vi "Handshake.vi"(8 "error in (no error)":errorcluster, 11 "dotNET SSL Socket in":refnum<class "dotNET SSL Server.lvclass">) -> (0 "error out":errorcluster, 3 "dotNET SSL Socket out":refnum<class "dotNET SSL Server.lvclass">)   [LabVIEW 2013, in "dotNET SSL Socket.lvlib" / "dotNET SSL Server.lvclass"]
uses:
  dotNET SSL Server/dotNET SSL Server.lvclass
  dotNET SSL Socket.lvclass/dotNET SSL Socket.ctl
  dotNET SSL Server/dotNET SSL Server.lvclass/dotNET SSL Server.ctl
  Read SSLStream.vi
  Read PFX Certificate.vi
  Read PFX Password.vi
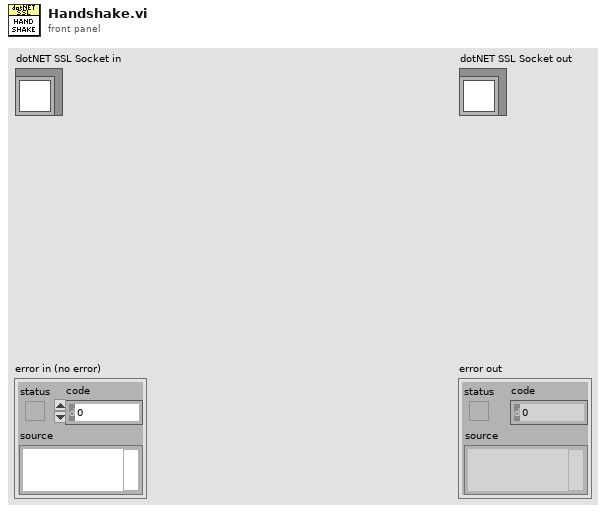
[diagram p1: front panel]
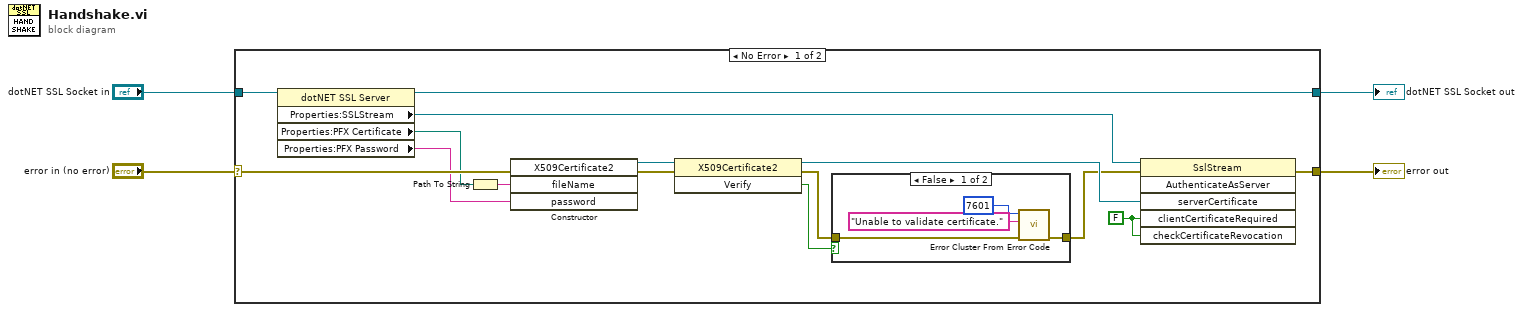
[diagram p0: block diagram]
diagram:
  n1 = case shown="No Error" "error in (no error)" {
    selector: "error in (no error)" -> [w15 w26]
    tunnel: [w18 w26] -> w3
    tunnel: [w5 w25] -> w1
    tunnel: "dotNET SSL Socket in" -> [w9 w25]
    frame No Error {
      w19 = FALSE ("clientCertificateRequired")
      n2 = property class="dotNET SSL Server"(reference=w9) -> (reference out=w5:refnum<class "dotNET SSL Server.lvclass">, "Properties:SSLStream"=w6:refnum<k24>, "Properties:PFX Certificate"=w8:path, "Properties:PFX Password"=w7:string)  [unwired: 1 in, 1 out]
      n3 = Path To String(path=w8) -> (string=w14:string)
      n4 = constructor class="X509Certificate2"(error in=w15, "fileName"=w14, "password"=w7) -> (reference out=w17:refnum<k24>, error out=w16:errorcluster)  [unwired: 2 in, 3 out]
      n5 = invoke class="X509Certificate2" method="Verify"(reference=w17, error in=w16) -> (reference out=w13:refnum<k24>, error out=w11:errorcluster, "Verify"=w12:bool)  [unwired: 1 in]
      n6 = case shown="False" w12 {
        tunnel: w11 -> [w22 w24]
        tunnel: [w23 w24] -> w10
        frame False {
          n7 = call <vilib>:"Error Cluster From Error Code.vi"("error in (no error)"=w22, "error message (\"\")"="Unable to validate certificate." ("error message (\"\")"), "error code (0)"=7601) -> ("error out"=w23:errorcluster)  [unwired: 6 in]
        }
        frame True {
        }
      }
      n8 = invoke class="SslStream" method="AuthenticateAsServer"(reference=w6, error in=w10, "serverCertificate"=w13, "clientCertificateRequired"=w19, "checkCertificateRevocation"=w19) -> (error out=w18:errorcluster)  [unwired: 1 in, 5 out]
    }
    frame Error {
    }
  }
  "error out" <- w3
  "dotNET SSL Socket out" <- w1
